vi "Run Shooter.vi"   [LabVIEW 2019]
uses:
  Robot Global Data.vi
types:
  T1 = typedef "WPI_MotorControlDeviceRef.ctl" = cluster{"DeviceStatus":errorcluster, "Type":T2, "PWM":cluster{"PWM Channel":T3, "DeadBand":T4}, "CAN":cluster{"Device Number":u8, "SetOutput VI Ref":variant, "GetOutput VI Ref":variant, "Enable VI Ref":variant, "Disable VI Ref":variant, "Data":variant}, "Invert":bool, "DIO PWM":cluster{"PWM \"Enable\" Channel":T3, "DIOChannel":T5, "PWM Rate":dbl}}
  T2 = typedef "WPI_MotorControlType.ctl" = enum16{"PWM", "CAN", "DIO PWM"}
  T3 = typedef "FPGA_DIOPWMChannel.ctl" = enum8{"PWM 0", "PWM 1", "PWM 2", "PWM 3", "PWM 4", "PWM 5", "PWM 6", "PWM 7", "PWM 8", "PWM 9", "PWM MXP 0", "PWM MXP 1", "PWM MXP 2", "PWM MXP 3", "PWM MXP 4", "PWM MXP 5", "PWM MXP 6", "PWM MXP 7", "PWM MXP 8", "PWM MXP 9", "Invalid"}
  T4 = typedef "WPI_PWMDeadband.ctl" = cluster{"Name":string, "maxPositivePwm":i32, "minPositivePwm":i32, "centerPwm":i32, "maxNegativePwm":i32, "minNegativePwm":i32, "angularRange":u16}
  T5 = typedef "FPGA_DIOChannel.ctl" = enum8{"DIO 0", "DIO 1", "DIO 2", "DIO 3", "DIO 4", "DIO 5", "DIO 6", "DIO 7", "DIO 8", "DIO 9", "DIO MXP 0", "DIO MXP 1", "DIO MXP 2", "DIO MXP 3", "DIO MXP 4", "DIO MXP 5", "DIO MXP 6", "DIO MXP 7", "DIO MXP 8", "DIO MXP 9", "DIO MXP 10", "DIO MXP 11", "DIO MXP 12", "DIO MXP 13", "DIO MXP 14", "DIO MXP 15", "SPI Port CS1", "SPI Port CS2", "SPI Port CS3", "SPI Port MISO", "SPI Port MOSI", "Invalid"}
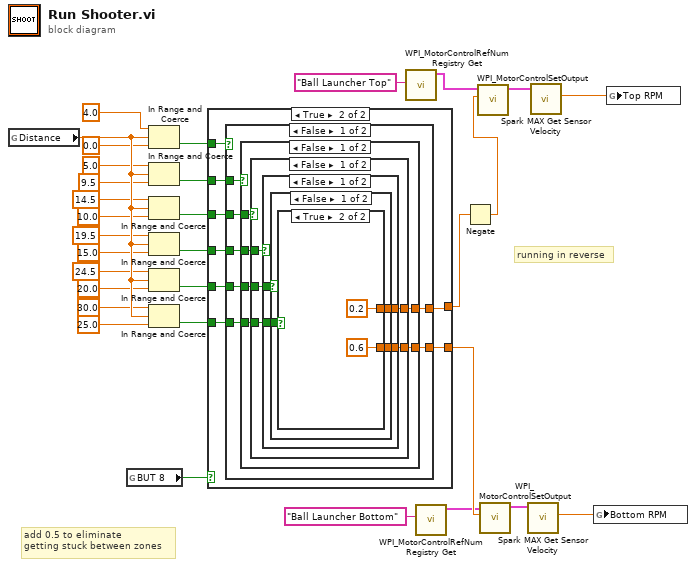
[diagram p0: block diagram]
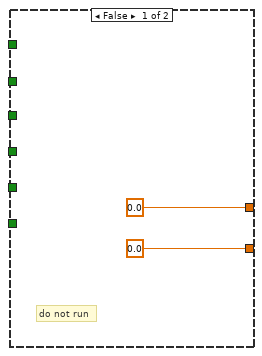
[diagram p2: hidden frame]
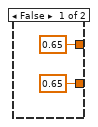
[diagram p3: hidden frame]
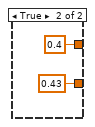
[diagram p4: hidden frame]
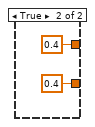
[diagram p5: hidden frame]
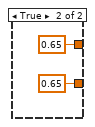
[diagram p6: hidden frame]
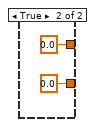
[diagram p7: hidden frame]
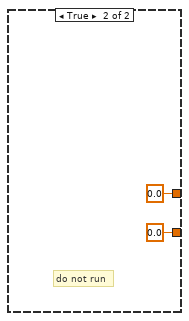
[diagram p8: hidden frame]
diagram:
  # "running in reverse"
  # "add 0.5 to eliminate\ngetting stuck between zones"
  n1 = global read "Robot Global Data.vi" "Distance"() -> (w31:dbl)
  n2 = global read "Robot Global Data.vi" "BUT 8"() -> (w9:bool)
  n3 = In Range and Coerce(upper limit=4.0, x=w31, lower limit=0.0) -> (In Range?=w28:bool)  [unwired: 1 out]
  n4 = In Range and Coerce(upper limit=5.0, x=w31, lower limit=9.5) -> (In Range?=w27:bool)  [unwired: 1 out]
  n5 = In Range and Coerce(upper limit=14.5, x=w31, lower limit=10.0) -> (In Range?=w11:bool)  [unwired: 1 out]
  n6 = In Range and Coerce(upper limit=19.5, x=w31, lower limit=15.0) -> (In Range?=w12:bool)  [unwired: 1 out]
  n7 = In Range and Coerce(upper limit=24.5, x=w31, lower limit=20.0) -> (In Range?=w13:bool)  [unwired: 1 out]
  n8 = In Range and Coerce(upper limit=30.0, x=w31, lower limit=25.0) -> (In Range?=w14:bool)  [unwired: 1 out]
  n9 = case shown="True" w9 {
    tunnel: [0.0 ("Output") w35] -> w30
    tunnel: [0.0 ("Output") w34] -> w10
    tunnel: w28 -> [_ w41]
    tunnel: w11 -> [_ w39]
    tunnel: w12 -> [_ w38]
    tunnel: w13 -> [_ w37]
    tunnel: w14 -> [_ w36]
    tunnel: w27 -> [_ w40]
    frame False {
      # "do not run"
    }
    frame True {
      n10 = case shown="False" w41 {
        tunnel: w40 -> [w48 _]
        tunnel: w39 -> [w47 _]
        tunnel: w38 -> [w46 _]
        tunnel: w37 -> [w45 _]
        tunnel: w36 -> [w44 _]
        tunnel: [w43 0.0 ("Output")] -> w35
        tunnel: [w42 0.0 ("Output")] -> w34
        frame False {
          n11 = case shown="False" w48 {
            tunnel: w47 -> [w54 _]
            tunnel: w46 -> [w53 _]
            tunnel: w45 -> [w52 _]
            tunnel: w44 -> [w51 _]
            tunnel: [w50 0.0 ("Output")] -> w43
            tunnel: [w49 0.0 ("Output")] -> w42
            frame False {
              n12 = case shown="False" w54 {
                tunnel: w53 -> [w59 _]
                tunnel: w52 -> [w58 _]
                tunnel: w51 -> [w57 _]
                tunnel: [w56 0.65 ("Output")] -> w50
                tunnel: [w55 0.65 ("Output")] -> w49
                frame False {
                  n13 = case shown="False" w59 {
                    tunnel: w58 -> [w63 _]
                    tunnel: w57 -> [w62 _]
                    tunnel: [w61 0.4 ("Output")] -> w56
                    tunnel: [w60 0.4 ("Output")] -> w55
                    frame False {
                      n14 = case shown="False" w63 {
                        tunnel: w62 -> [w66 _]
                        tunnel: [w65 0.4 ("Output")] -> w61
                        tunnel: [w64 0.43 ("Output")] -> w60
                        frame False {
                          n15 = case shown="True" w66 {
                            tunnel: [0.65 ("Output") 0.2 ("Output")] -> w65
                            tunnel: [0.65 ("Output") 0.6 ("Output")] -> w64
                            frame False {
                            }
                            frame True {
                            }
                          }
                        }
                        frame True {
                        }
                      }
                    }
                    frame True {
                    }
                  }
                }
                frame True {
                }
              }
            }
            frame True {
            }
          }
        }
        frame True {
          # "do not run"
        }
      }
    }
  }
  n16 = call <vilib>:"WPI_MotorControlRefNum Registry Get.vi"("refnum name"="Ball Launcher Top") -> ("MotorControlDevRef"=w4:T1)  [unwired: 9 in, 1 out]
  n17 = call <vilib>:"WPI_MotorControlRefNum Registry Get.vi"("refnum name"="Ball Launcher Bottom") -> ("MotorControlDevRef"=w2:T1)  [unwired: 9 in, 1 out]
  n18 = Negate(x=w30) -> (-x=w29:dbl)
  n19 = call <vilib>:"WPI_MotorControlSetOutput.vi"("Output"=w29, "MotorControlDevRef"=w4) -> ("MotorControlDevRef"=w7:T1)  [unwired: 7 in, 2 out]
  n20 = call <vilib>:"WPI_MotorControlSetOutput.vi"("Output"=w10, "MotorControlDevRef"=w2) -> ("MotorControlDevRef"=w8:T1)  [unwired: 7 in, 2 out]
  n21 = call <vilib>:"Spark MAX Get Sensor Velocity.vi"("MotorControlDevRef in"=w8) -> ("Sensor Velocity"=w6:dbl)  [unwired: 7 in, 3 out]
  n22 = call <vilib>:"Spark MAX Get Sensor Velocity.vi"("MotorControlDevRef in"=w7) -> ("Sensor Velocity"=w5:dbl)  [unwired: 7 in, 3 out]
  n23 = global write "Robot Global Data.vi" "Bottom RPM"(w6) -> ()
  n24 = global write "Robot Global Data.vi" "Top RPM"(w5) -> ()
